vi "Receive Message.vi"(8 "error in (no error)":errorcluster, 10 "timeout ms":i32=-1, 11 "Stream in":refnum<class "Stream.lvclass">) -> (0 "error out":errorcluster, 3 "Stream out":refnum<class "Stream.lvclass">)   [LabVIEW 2018, in "Stream.lvclass"]
uses:
  Stream.lvclass
  Stream.lvclass/Stream.ctl
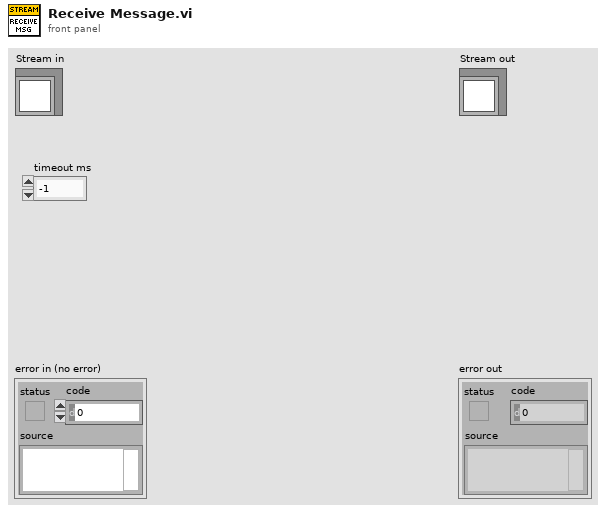
[diagram p1: front panel]
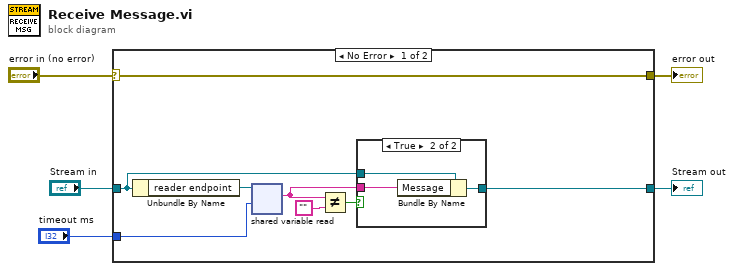
[diagram p0: block diagram]
diagram:
  n1 = case shown="No Error" "error in (no error)" {
    selector: "error in (no error)" -> [w10 w19]
    tunnel: [w10 w19] -> w4
    tunnel: [w11 w18] -> w3
    tunnel: "Stream in" -> [w12 w18]
    tunnel: "timeout ms" -> [w6 _]
    frame No Error {
      n2 = Unbundle By Name(w12) -> ("reader endpoint"=w13:refnum<k21>)
      n3 = shared-variable-read(w13, w6) -> (w9:string)  [unwired: 1 in, 3 out]
      n4 = Not Equal?(x=w9, y="") -> (x != y?=w7:bool)
      n5 = case shown="True" w7 {
        tunnel: w9 -> [_ w17]
        tunnel: w12 -> [w14 w16]
        tunnel: [w14 w15] -> w11
        frame False {
        }
        frame True {
          n6 = Bundle By Name(cluster=w16, "Message"=w17) -> (w15:refnum<class "Stream.lvclass">)
        }
      }
    }
    frame Error {
    }
  }
  "error out" <- w4
  "Stream out" <- w3
